vi "Measure.vi"(8 "error in (no error)":errorcluster, 11 "EpiWrapper in":refnum<class "EpiWrapper.lvclass">) -> (0 "error out":errorcluster, 3 "EpiWrapper out":refnum<class "EpiWrapper.lvclass">)   [LabVIEW 2012, in "EpiWrapper.lvclass"]
uses:
  EpiWrapper.lvclass
  EpiWrapper.lvclass/EpiWrapper.ctl
  Instruments.lvclass
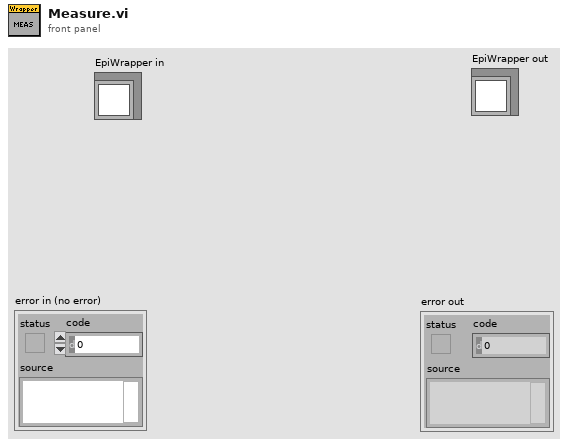
[diagram p1: front panel]
types:
  T1 = typedef "CurrentPad.ctl" = cluster{"Coords":cluster{"Horizontal":sgl, "Vertical":sgl}, "radius":i32, "Tested":bool, "Selected":bool, "Pad":string, "PadArea":T2}
  T2 = typedef "PadArea.ctl" = enum16{"A", "B", "C", "D", "L", "R", "T", "G"}
  T3 = typedef "TestData.ctl" = cluster{"20mA Data":T4, "50mA Data ":T4}
  T4 = typedef "Measurement.ctl" = cluster{"Area":string, "Pad":string, "Current,mA":dbl, "Power":dbl, "WL":dbl, "Voltage":dbl, "Knee Current":dbl, "Reverse":dbl}
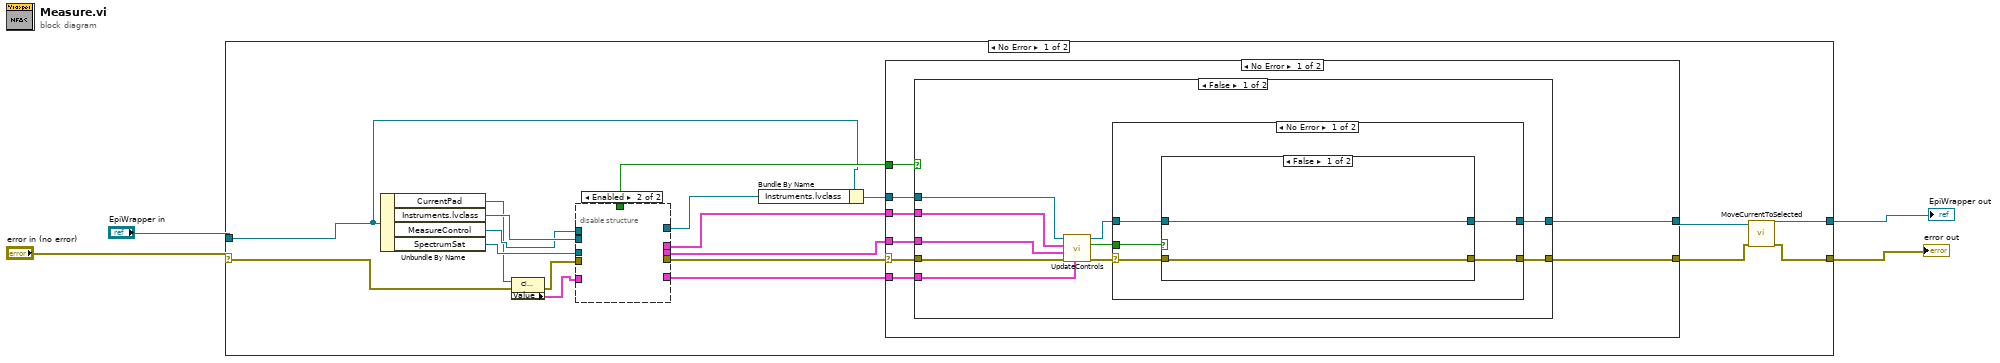
[diagram p0: block diagram]
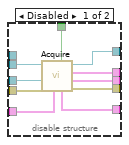
[diagram p2: hidden frame]
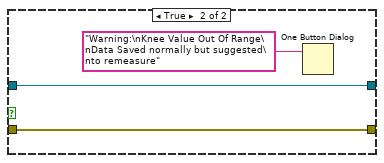
[diagram p3: hidden frame]
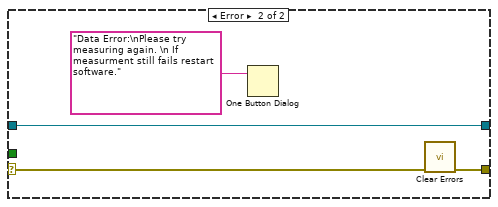
[diagram p4: hidden frame]
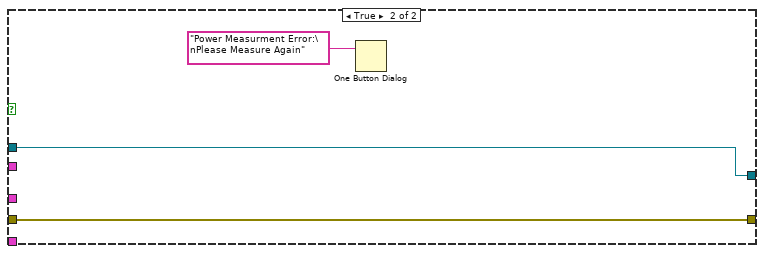
[diagram p5: hidden frame]
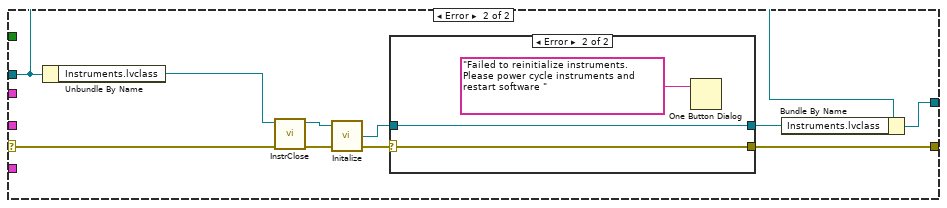
[diagram p6: hidden frame]
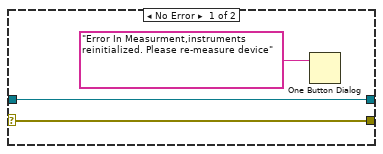
[diagram p7: hidden frame]
diagram:
  n1 = case shown="No Error" "error in (no error)" {
    selector: "error in (no error)" -> [w7 w86]
    tunnel: [w11 w86] -> w2
    tunnel: [w10 w85] -> w1
    tunnel: "EpiWrapper in" -> [w14 w85]
    frame No Error {
      n2 = Unbundle By Name(w14) -> ("CurrentPad"=w8:refnum<vi>, "Instruments.lvclass"=w23:refnum<class "Instruments.lvclass">, "MeasureControl"=w9:refnum<vi>, "SpectrumSat"=w15:refnum<vi>)
      n3 = property class="Clust (strict)"(reference=w8, error in=w7) -> (error out=w6:errorcluster, "Value"=w5:T1)  [unwired: 1 out]
      n4 = disable-structure shown="Enabled" {
        disable-tunnel: w23 -> [w33 _]
        disable-tunnel: [w32 _] -> w22
        disable-tunnel: [w31 _] -> w20
        disable-tunnel: [w30 _] -> w19
        disable-tunnel: [w29 _] -> w18
        disable-tunnel: [w28 _] -> w17
        disable-tunnel: [w27 _] -> w16
        disable-tunnel: w15 -> [w26 _]
        disable-tunnel: w6 -> [w25 _]
        disable-tunnel: w9 -> [_ _]
        disable-tunnel: w5 -> [w24 _]
        frame Disabled {
          n5 = call-dynamic "Acquire.vi"("CurrentPad"=w24, "error in (no error)"=w25, "SpectrumSat"=w26, "Instruments in"=w33) -> ("error out"=w27:errorcluster, "20mA Spectra"=w30:cluster{"Wavelength":dbl[], "EL Spectrum":dbl[]}, "Data Out"=w28:T3, "Instruments out"=w32:refnum<class "Instruments.lvclass">, "50mA Spectra"=w29:cluster{"Wavelength":dbl[], "EL Spectrum":dbl[]}, "remeasure?"=w31:bool)  [unwired: 2 in]
        }
        frame Enabled {
        }
      }
      n6 = Bundle By Name(cluster=w14, "Instruments.lvclass"=w22) -> (w21:refnum<class "EpiWrapper.lvclass">)
      n7 = case shown="No Error" w16 {
        selector: w16 -> [w34 w71]
        tunnel: w21 -> [w41 w75]
        tunnel: w20 -> [w40 _]
        tunnel: [w39 w73] -> w13
        tunnel: [w38 w76] -> w12
        tunnel: w19 -> [w37 _]
        tunnel: w18 -> [w36 _]
        tunnel: w17 -> [w35 _]
        frame No Error {
          n8 = case shown="False" w40 {
            tunnel: w35 -> [w51 _]
            tunnel: w41 -> [w50 w66]
            tunnel: [w45 w66] -> w39
            tunnel: [w44 w67] -> w38
            tunnel: w34 -> [w43 w67]
            tunnel: w37 -> [w49 _]
            tunnel: w36 -> [w48 _]
            frame False {
              n9 = call-dynamic "UpdateControls.vi"("50mA Spectra"=w48, "error in (no error)"=w43, "20mA Spectra"=w49, "Data In"=w51, "EpiWrapper in"=w50) -> ("error out"=w47:errorcluster, "KneeFail?"=w42:bool, "EpiWrapper out"=w46:refnum<class "EpiWrapper.lvclass">)  [unwired: 4 in]
              n10 = case shown="No Error" w47 {
                selector: w47 -> [w54 w65]
                tunnel: w46 -> [w53 w62]
                tunnel: [w52 w62] -> w45
                tunnel: [w55 w63] -> w44
                tunnel: w42 -> [w56 _]
                frame No Error {
                  n11 = case shown="False" w56 {
                    tunnel: [w57 w60] -> w55
                    tunnel: w54 -> [w57 w60]
                    tunnel: w53 -> [w58 w59]
                    tunnel: [w58 w59] -> w52
                    frame False {
                    }
                    frame True {
                      n12 = One Button Dialog(message="Warning:\nKnee Value Out Of Range\nData Saved normally but suggested\nto remeasure") -> ()  [unwired: 1 in, 1 out]
                    }
                  }
                }
                frame Error {
                  n13 = One Button Dialog(message="Data Error:\nPlease try measuring again. \n If measurment still fails restart software.") -> ()  [unwired: 1 in, 1 out]
                  n14 = call <vilib>:"Clear Errors.vi"("error in (no error)"=w65) -> ("error out"=w63:errorcluster)  [unwired: 6 in]
                }
              }
            }
            frame True {
              n15 = One Button Dialog(message="Power Measurment Error:\nPlease Measure Again") -> ()  [unwired: 1 in, 1 out]
            }
          }
        }
        frame Error {
          n16 = Unbundle By Name(w75) -> ("Instruments.lvclass"=w70:refnum<class "Instruments.lvclass">)
          n17 = call-dynamic "InstrClose.vi"("error in (no error)"=w71, "Instruments in"=w70) -> ("error out"=w72:errorcluster, "Instruments out"=w69:refnum<class "Instruments.lvclass">)  [unwired: 8 in]
          n18 = call-dynamic "Initalize.vi"("error in (no error)"=w72, "Instruments in"=w69) -> ("error out"=w78:errorcluster, "Instruments out"=w77:refnum<class "Instruments.lvclass">)  [unwired: 2 in]
          n19 = case shown="Error" w78 {
            selector: w78 -> [w79 w82]
            tunnel: w77 -> [w80 w83]
            tunnel: [w80 w83] -> w74
            tunnel: [w79 w82] -> w76
            frame No Error {
              n20 = One Button Dialog(message="Error In Measurment,instruments reinitialized. Please re-measure device") -> ()  [unwired: 1 in, 1 out]
            }
            frame Error {
              n21 = One Button Dialog(message="Failed to reinitialize instruments.  Please power cycle instruments and restart software ") -> ()  [unwired: 1 in, 1 out]
            }
          }
          n22 = Bundle By Name(cluster=w75, "Instruments.lvclass"=w74) -> (w73:refnum<class "EpiWrapper.lvclass">)
        }
      }
      n23 = call-dynamic "MoveCurrentToSelected.vi"("error in (no error)"=w12, "EpiWrapper in"=w13) -> ("error out"=w11:errorcluster, "EpiWrapper out"=w10:refnum<class "EpiWrapper.lvclass">)  [unwired: 8 in]
    }
    frame Error {
    }
  }
  "error out" <- w2
  "EpiWrapper out" <- w1
